vi "Wait for Deposit.vi"(8 "错误输入":errorcluster, 11 "帐户信息":T1) -> (0 "错误输出":errorcluster, 1 "停止？":bool, 2 "存款额":dbl, 3 "帐户信息输出":T1)   [LabVIEW 2012]
uses:
  Account Info.ctl
  Stop.vi
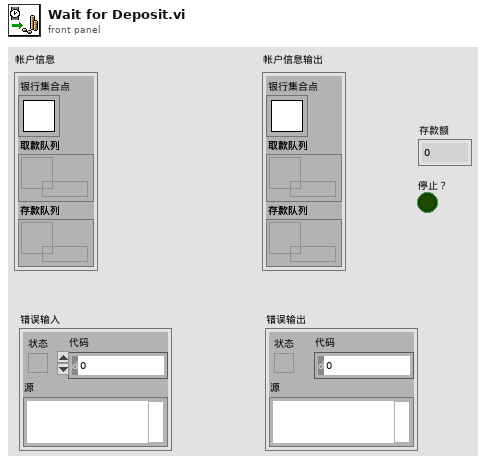
[diagram p1: front panel]
types:
  T1 = typedef "Account Info.ctl" = cluster{"银行集合点":T2, "取款队列":refnum<queue>, "存款队列":refnum<queue>}
  T2 = typedef "Rendezvous RefNum" = refnum<k1>
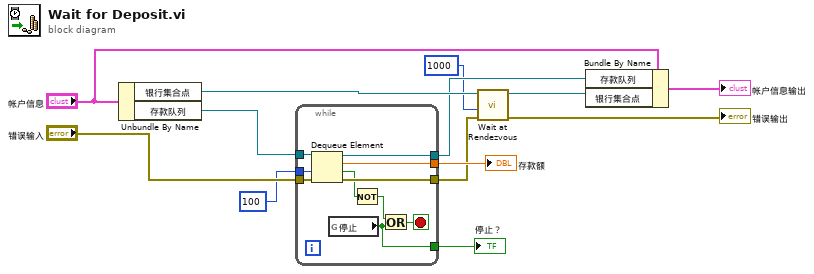
[diagram p0: block diagram]
diagram:
  n1 = Unbundle By Name ("按名称解除捆绑")("帐户信息") -> ("银行集合点"=w10:T2, "存款队列"=w13:refnum<queue>)
  n2 = while {
    tunnel: w13 -> [w23]
    tunnel: [w22] -> w12
    tunnel: "错误输入" -> [w21]
    tunnel: [w20] -> w9
    tunnel: [w19] -> w6
    tunnel: 100 ("超时毫秒(-1)") -> [w15]
    tunnel: [w14] -> w1
    stop <- w18 stop-if-true
    n3 = Dequeue Element ("元素出队列")(queue=w23, timeout in ms (-1)=w15, error in (no error)=w21) -> (queue out=w19:refnum<queue>, element=w22:dbl, timed out?=w16:bool, error out=w20:errorcluster)
    n4 = global read "Stop.vi" "停止"() -> (w14:bool)
    n5 = Not ("非")(x=w16) -> (.not. x?=w17:bool)
    n6 = Or ("或")(x=w17, y=w14) -> (x .or. y?=w18:bool)
  }
  "存款额" <- w12
  "停止？" <- w1
  n7 = call <vilib>:"Wait at Rendezvous.vi"("error in (no error)"=w9, "ms timeout (-1)"=1000 ("毫秒超时(-1)"), "rendezvous"=w10) -> ("error out"=→"错误输出":errorcluster, "rendezvous out"=w7:T2)  [unwired: 2 in, 1 out]
  n8 = Bundle By Name ("按名称捆绑")(cluster="帐户信息", "存款队列"=w6, "银行集合点"=w7) -> (→"帐户信息输出":T1)
